vi "DI Redraw Boost Slider.vi"(7 "Bank A? (T)":bool=TRUE, 8 "DCM System State":T3 {"System ADC"."Fan [V]" format="%#_3p"; "System ADC"."Primary B1B2 [V]" format="%#_3p"; "System ADC"."Primary B3B4 [V]" format="%#_3p"; "System ADC"."Primary A3A4 [V]" format="%#_3p"; "System ADC"."Primary A1A2 [V]" format="%#_3p"; "System ADC"."MPRD [V]" format="%#_3p"; "System ADC"."Ext HV B [V]" format="%#_3p"; "System ADC"."Ext HV A [V]" format="%#_3p"; "System ADC"."Pump Zener B [V]" format="%#_3p"; "System ADC"."Pump Zener A [V]" format="%#_3p"; "System ADC"."DI Zener B [V]" format="%#_3p"; "System ADC"."DI Zener A [V]" format="%#_3p"; "System ADC"."Key [V]" format="%#_3p"; "System ADC"."DRVP [V]" format="%#_3p"; "System ADC"."Battery [V]" format="%#_3p"; "System ADC"."FET Driver [V]" format="%#_3p"; "System ADC"."Secondary B1B2 [V]" format="%#_3p"; "System ADC"."Secondary B3B4 [V]" format="%#_3p"; "System ADC"."Secondary A3A4 [V]" format="%#_3p"; "System ADC"."Secondary A1A2 [V]" format="%#_3p"; "System ADC"."Primary Range [V]" format="%#_3p"; "System ADC"."Temp Boost B [C]" format="%#_3p"; "System ADC"."Temp Primary A [C]" format="%#_3p"; "System ADC"."Temp Secondary A [C]" format="%#_3p"; "System ADC"."Temp Fan Intake [C]" format="%#_3p"; "System ADC"."Temp CPU [C]" format="%#_3p"; "System ADC"."Temp DI Zener B [C]" format="%#_3p"; "System ADC"."Temp DI B [C]" format="%#_3p"; "System ADC"."Temp DI Zener A [C]" format="%#_3p"; "System ADC"."Temp DI A [C]" format="%#_3p"; "System ADC"."Temp HH 7-12 [C]" format="%#_3p"; "System ADC"."Temp HH 1-6 [C]" format="%#_3p"; "System ADC"."AI 12 [V]" format="%#_3p"; "System ADC"."AI 11 [V]" format="%#_3p"; "System ADC"."AI 10 [V]" format="%#_3p"; "System ADC"."AI 9 [V]" format="%#_3p"; "System ADC"."AI 8 [V]" format="%#_3p"; "System ADC"."AI 7 [V]" format="%#_3p"; "System ADC"."AI 6 [V]" format="%#_3p"; "System ADC"."AI 5 [V]" format="%#_3p"; "System ADC"."AI 4 [V]" format="%#_3p"; "System ADC"."AI 3 [V]" format="%#_3p"; "System ADC"."AI 2 [V]" format="%#_3p"; "System ADC"."AI 1 [V]" format="%#_3p"}, 11 "DI Bank Configuration":T1 caption="Configuration" {"Pump Zener Voltage [V]" min=0 max=240 format="%#_13g"; "DI Zener Voltage [V]" min=0 max=100 format="%#_13g"; "Boost Clamp [V]" min=0 max=220 format="%#_13g"; "Boost Voltage [V]" min=0 max=220 format="%#_13g"}) -> (3 "Levels Slider":cluster{dbl, dbl, dbl, dbl}(slide)={0.0, 0.0, 14.742268041237113, 14.742268041237113} scale=0.0..220.0)   [LabVIEW 2016]
uses:
  <vilib>/Powertrain Controls/Device Drivers/DCM/Rev0/RT/System State.ctl
  <vilib>/Powertrain Controls/Device Drivers/DCM/Rev0/RT/System ADC.ctl
  <vilib>/Powertrain Controls/Device Drivers/DCM/Rev0/RT/Internal Fault.ctl
  <vilib>/Powertrain Controls/Device Drivers/DCM/Rev0/RT/Configuration.ctl
  <vilib>/Powertrain Controls/Device Drivers/DCM/Rev0/FPGA/DI - Bank Configuration.ctl
  <vilib>/Powertrain Controls/Device Drivers/DCM/Rev0/RT/DCM - RT.lvclass
  <vilib>/Powertrain Controls/Device Drivers/DCM/Rev0/FPGA/DCM - FPGA.lvlib
panel:
  # "DI Backboost"
  # "Pump Backboost"
  # "High Voltage"
  # "Boost Clamp"
  # "Voltage [DV]"
  # "Voltage [V]"
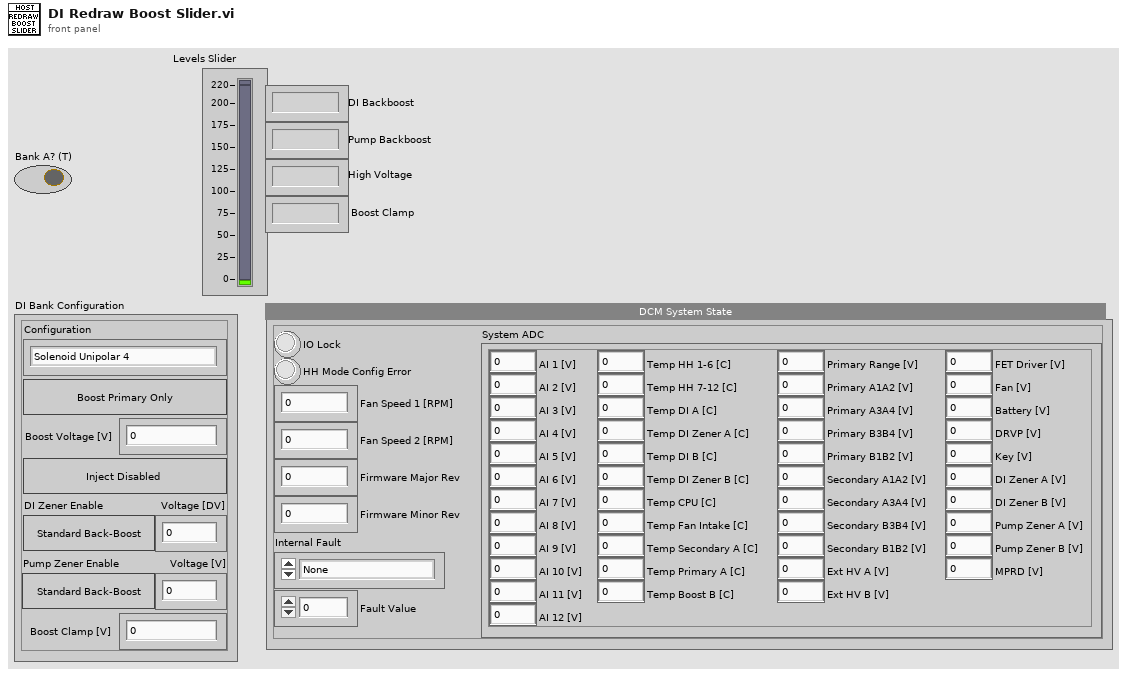
[diagram p1: front panel]
types:
  T1 = typedef "DCM - RT.lvclass/Configuration.ctl" = cluster{"Configuration":T2, "Power Supply Enable":bool, "Boost Voltage [V]":sgl, "Inject Enable":bool, "DI Zener Enable":bool, "DI Zener Voltage [V]":sgl, "Pump Zener Enable":bool, "Pump Zener Voltage [V]":sgl, "Boost Clamp [V]":sgl}
  T2 = typedef "DCM - FPGA.lvlib/DI - Bank Configuration.ctl" = enum8{"Solenoid Unipolar 4", "Solenoid Unipolar 7 (Muxed)", "Solenoid Unipolar 8 (Muxed)", "Solenoid Bipolar 2", "Solenoid Bipolar 3 (Muxed)", "Piezo Unipolar 2", "Piezo Unipolar 3 (Muxed)", "Piezo Unipolar 4 (Muxed)", "Piezo Bipolar 2", "Piezo Bipolar 3 (Muxed)"}
  T3 = typedef "DCM - RT.lvclass/System State.ctl" = cluster{"System ADC":T4, "IO Lock":bool, "HH Mode Config Error":bool, "Fan Speed 1 [RPM]":sgl, "Fan Speed 2 [RPM]":sgl, "Firmware Major Rev":u16, "Firmware Minor Rev":u16, "Internal Fault":T5, "Fault Value":dbl}
  T4 = typedef "DCM - RT.lvclass/System ADC.ctl" = cluster{"AI 1 [V]":sgl, "AI 2 [V]":sgl, "AI 3 [V]":sgl, "AI 4 [V]":sgl, "AI 5 [V]":sgl, "AI 6 [V]":sgl, "AI 7 [V]":sgl, "AI 8 [V]":sgl, "AI 9 [V]":sgl, "AI 10 [V]":sgl, "AI 11 [V]":sgl, "AI 12 [V]":sgl, "Temp HH 1-6 [C]":sgl, "Temp HH 7-12 [C]":sgl, "Temp DI A [C]":sgl, "Temp DI Zener A [C]":sgl, "Temp DI B [C]":sgl, "Temp DI Zener B [C]":sgl, "Temp CPU [C]":sgl, "Temp Fan Intake [C]":sgl, "Temp Secondary A [C]":sgl, "Temp Primary A [C]":sgl, "Temp Boost B [C]":sgl, "Primary Range [V]":sgl, "Primary A1A2 [V]":sgl, "Primary A3A4 [V]":sgl, "Primary B3B4 [V]":sgl, "Primary B1B2 [V]":sgl, "Secondary A1A2 [V]":sgl, "Secondary A3A4 [V]":sgl, "Secondary B3B4 [V]":sgl, "Secondary B1B2 [V]":sgl, "Ext HV A [V]":sgl, "Ext HV B [V]":sgl, "FET Driver [V]":sgl, "Fan [V]":sgl, "Battery [V]":sgl, "DRVP [V]":sgl, "Key [V]":sgl, "DI Zener A [V]":sgl, "DI Zener B [V]":sgl, "Pump Zener A [V]":sgl, "Pump Zener B [V]":sgl, "MPRD [V]":sgl}
  T5 = typedef "DCM - RT.lvclass/Internal Fault.ctl" = enum32{"None", "Temp HH 1-6", "Temp HH 7-12", "Temp DI A", "Temp DI Zener A", "Temp DI B", "Temp DI Zener B", "Temp Intake", "Temp Primary A", "Temp Secondary A", "Temp Boost B", "Temp CPU", "Low Battery", "Inrush Protection", "A Run Enable", "B Run Enable"}
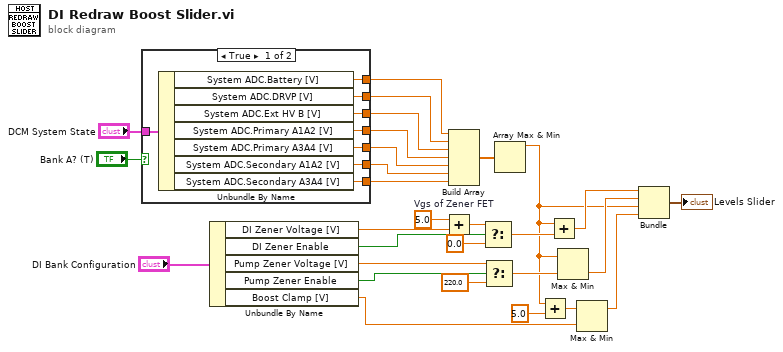
[diagram p0: block diagram]
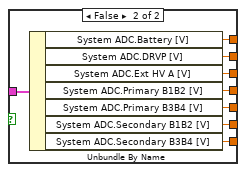
[diagram p2: hidden frame]
diagram:
  w13 = 5.0  # Vgs of Zener FET
  n1 = case shown="True" "Bank A? (T)" {
    tunnel: "DCM System State" -> [w37 w45]
    tunnel: [w36 w44] -> w26
    tunnel: [w35 w43] -> w25
    tunnel: [w34 w42] -> w6
    tunnel: [w33 w41] -> w5
    tunnel: [w32 w40] -> w4
    tunnel: [w31 w39] -> w3
    tunnel: [w30 w38] -> w2
    frame True {
      n2 = Unbundle By Name(w37) -> ("System ADC.Battery [V]"=w36:sgl, "System ADC.DRVP [V]"=w35:sgl, "System ADC.Ext HV B [V]"=w34:sgl, "System ADC.Primary A1A2 [V]"=w33:sgl, "System ADC.Primary A3A4 [V]"=w32:sgl, "System ADC.Secondary A1A2 [V]"=w31:sgl, "System ADC.Secondary A3A4 [V]"=w30:sgl)
    }
    frame False {
      n3 = Unbundle By Name(w45) -> ("System ADC.Battery [V]"=w44:sgl, "System ADC.DRVP [V]"=w43:sgl, "System ADC.Ext HV A [V]"=w42:sgl, "System ADC.Primary B1B2 [V]"=w41:sgl, "System ADC.Primary B3B4 [V]"=w40:sgl, "System ADC.Secondary B1B2 [V]"=w39:sgl, "System ADC.Secondary B3B4 [V]"=w38:sgl)
    }
  }
  n4 = Unbundle By Name("DI Bank Configuration") -> ("DI Zener Voltage [V]"=w24:sgl, "DI Zener Enable"=w23:bool, "Pump Zener Voltage [V]"=w22:sgl, "Pump Zener Enable"=w21:bool, "Boost Clamp [V]"=w10:sgl)
  n5 = Add(x=w13, y=w24) -> (x+y=w14:dbl)
  n6 = Build Array(w26, w25, w6, w5, w4, w3, w2) -> (w20:sgl[])
  n7 = Select(t=w14, s=w23, f=0.0) -> (s? t:f=w16:dbl)
  n8 = Select(t=w22, s=w21, f=220.0) -> (s? t:f=w12:dbl)
  n9 = Array Max & Min(array=w20) -> (max value=w7:sgl)  [unwired: 3 out]
  n10 = Add(x=w7, y=5.0) -> (x+y=w18:dbl)
  n11 = Add(x=w7, y=w16) -> (x+y=w9:dbl)
  n12 = Max & Min(x=w7, y=w12) -> (min(x,y)=w8:dbl)  [unwired: 1 out]
  n13 = Max & Min(x=w18, y=w10) -> (max(x,y)=w11:dbl)  [unwired: 1 out]
  n14 = Bundle(w9, w8, w7, w11) -> (→"Levels Slider":cluster{dbl, dbl, sgl, dbl})  [unwired: 1 in]
